vi "SSL Detection Frame.vi"(8 "error in":errorcluster, 9 "Array":u8[](array[numeric]) format="%02x") -> (0 "error out":errorcluster, 3 "Detection Frame":T1)   [LabVIEW 2016]
uses:
  SSL Detection Frame.ctl
  SSL Detection Robot.ctl
  SSL Detection Ball.ctl
  Varint Decoder uint32.vi
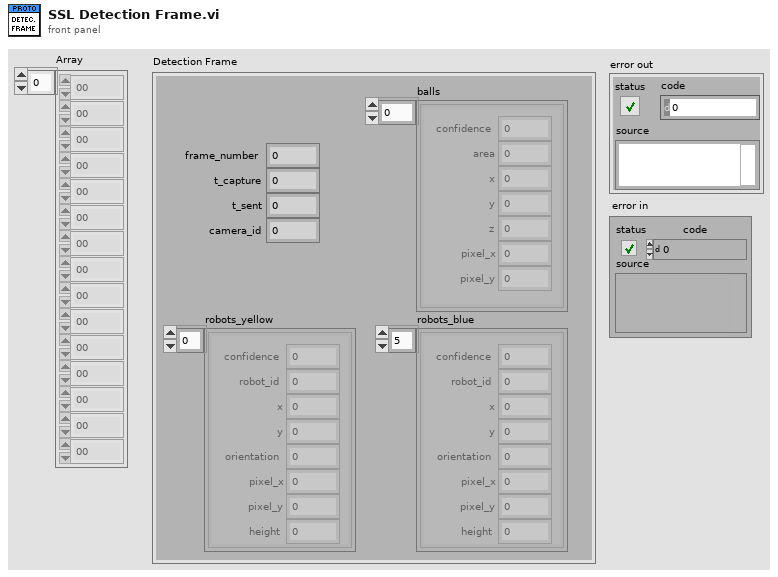
[diagram p1: front panel]
types:
  T1 = typedef "SSL Detection Frame.ctl" = cluster{"frame_number":u32, "t_capture":dbl, "t_sent":dbl, "camera_id":u32, "robots_yellow":T2[], "robots_blue":T2[], "balls":T3[]}
  T2 = typedef "SSL Detection Robot.ctl" = cluster{"x":dbl, "robot_id":u32, "confidence":sgl, "y":sgl, "orientation":sgl, "pixel_x":sgl, "pixel_y":sgl, "height":sgl}
  T3 = typedef "SSL Detection Ball.ctl" = cluster{"x":sgl, "area":u32, "confidence":sgl, "y":sgl, "z":sgl, "pixel_x":sgl, "pixel_y":sgl}
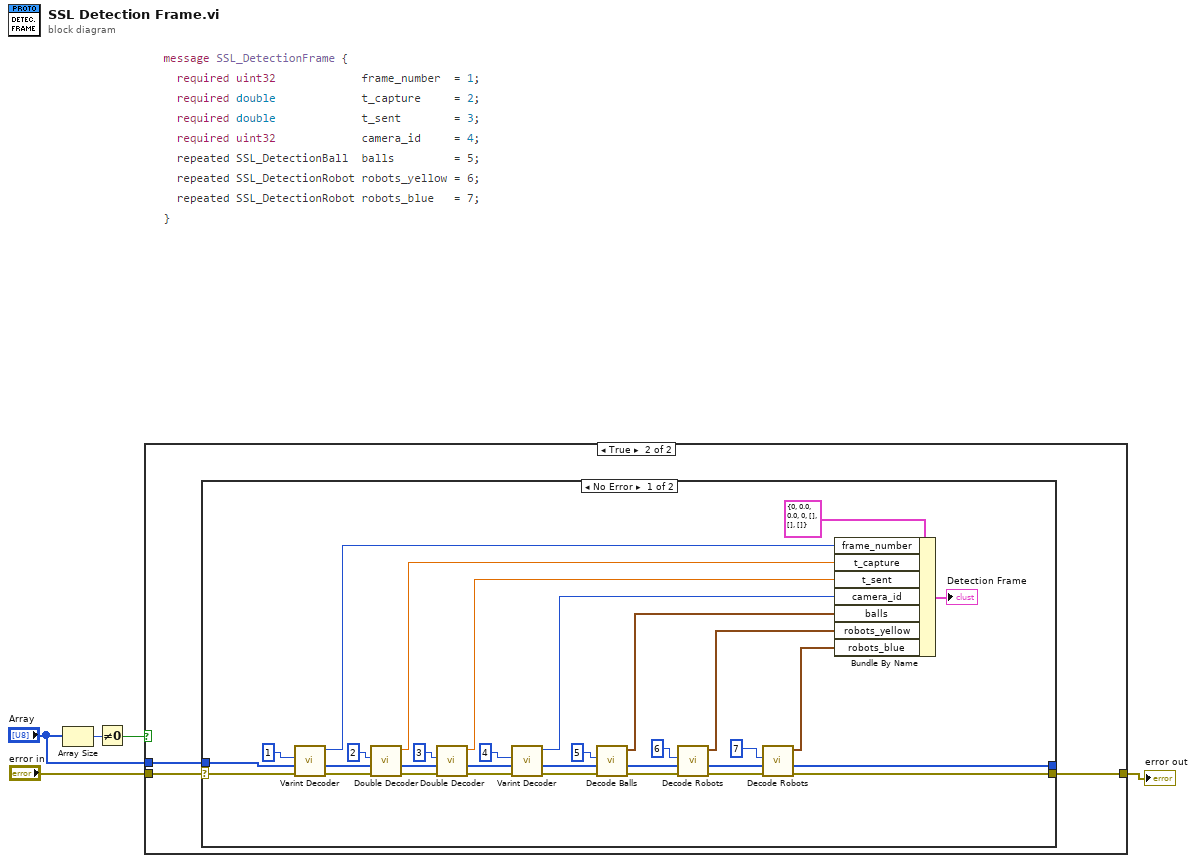
[diagram p0: block diagram]
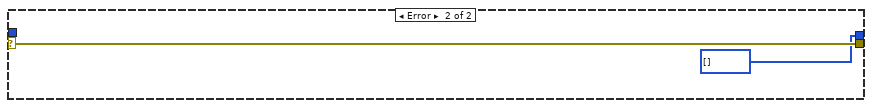
[diagram p3: hidden frame]
diagram:
  n1 = Array Size(array="Array") -> (size(s)=w3:i32)
  n2 = Not Equal To 0?(x=w3) -> (x != 0?=w1:bool)
  n3 = case shown="True" w1 {
    tunnel: "error in" -> [_ w8]
    tunnel: "Array" -> [_ w7]
    tunnel: [_ w6] -> w2
    frame False {
    }
    frame True {
      n4 = case shown="No Error" w8 {
        selector: w8 -> [w39 w42]
        tunnel: [w10 w42] -> w6
        tunnel: [w11 u8[] [] ("array w/ subset deleted")] -> _
        tunnel: w7 -> [w9 _]
        frame No Error {
          n5 = call-poly "Varint Decoder.vi"("error in (no error)"=w39, "Array"=w9, "Key"=1) -> ("error out"=w38:errorcluster, "array w/ subset deleted"=w21:u8[], "Varint"=w27:u32)  [unwired: 5 in, 1 out]
          n6 = call "Double Decoder.vi"("error in (no error)"=w38, "Array"=w21, "Key"=2) -> ("error out"=w37:errorcluster, "array w/ subset deleted"=w22:u8[], "Double"=w28:dbl)  [unwired: 5 in, 1 out]
          n7 = call "Double Decoder.vi"("error in (no error)"=w37, "Array"=w22, "Key"=3) -> ("error out"=w36:errorcluster, "array w/ subset deleted"=w23:u8[], "Double"=w29:dbl)  [unwired: 5 in, 1 out]
          n8 = call-poly "Varint Decoder.vi"("error in (no error)"=w36, "Array"=w23, "Key"=4) -> ("error out"=w32:errorcluster, "array w/ subset deleted"=w24:u8[], "Varint"=w30:u32)  [unwired: 5 in, 1 out]
          n9 = call "Decode Balls.vi"("error in"=w32, "array"=w24, "Key"=5) -> ("error out"=w19:errorcluster, "array w/ subset deleted out"=w18:u8[], "Array"=w25:T3[])  [unwired: 6 in]
          n10 = call "Decode Robots.vi"("error in"=w19, "array"=w18, "Key"=6) -> ("error out"=w16:errorcluster, "array w/ subset deleted out"=w15:u8[], "Robots"=w13:T2[])  [unwired: 6 in]
          n11 = call "Decode Robots.vi"("error in"=w16, "array"=w15, "Key"=7) -> ("error out"=w10:errorcluster, "array w/ subset deleted out"=w11:u8[], "Robots"=w12:T2[])  [unwired: 6 in]
          n12 = Bundle By Name(cluster=T1 {"frame_number"=0, "t_capture"=0.0, "t_sent"=0.0, "camera_id"=0, "robots_yellow"=[], "robots_blue"=[], "balls"=[]} ("Detection Frame 2"), "frame_number"=w27, "t_capture"=w28, "t_sent"=w29, "camera_id"=w30, "balls"=w25, "robots_yellow"=w13, "robots_blue"=w12) -> (→"Detection Frame":T1)
        }
        frame Error {
        }
      }
    }
  }
  "error out" <- w2
